vi "Evaluate Part 2.vi"() -> ()   [LabVIEW 2021]
uses:
  Race/Race.lvclass
panel:
  in  "Distance":u64=940200
  in  "Time":u64=71530
  out "Ways to Win":u64=71503
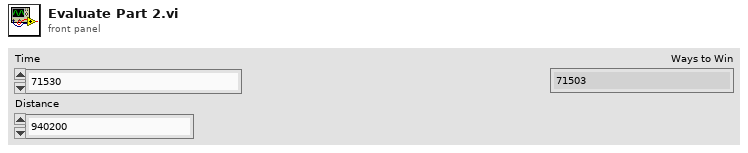
[diagram p1: front panel]
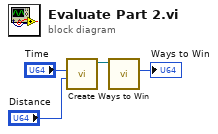
[diagram p0: block diagram]
diagram:
  n1 = call "Create.vi"("Distance"="Distance", "Time"="Time") -> ("Race Out"=w4:refnum<class "Race.lvclass">)  [unwired: 8 in, 1 out]
  n2 = call "Ways to Win.vi"("Race In"=w4) -> ("Ways to win"=→"Ways to Win":u64)  [unwired: 9 in, 1 out]
